vi "Profile Descriptor.vi"(10 "Profile":string[](array[string]), 11 "Descriptor":string) -> (3 "Flavoured Descriptor":string)   [LabVIEW 2015]
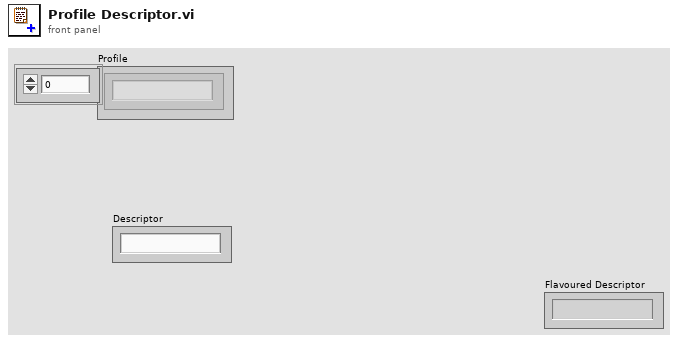
[diagram p1: front panel]
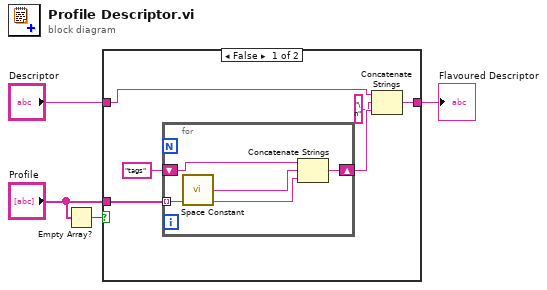
[diagram p0: block diagram]
diagram:
  n1 = Empty Array?(array="Profile") -> (empty?=w1:bool)
  n2 = case shown="False" w1 {
    tunnel: "Profile" -> [w10 _]
    tunnel: "Descriptor" -> [w9 w15]
    tunnel: [w8 w15] -> w3
    frame False {
      n3 = for {
        tunnel: w10 -> [w11] mode=indexing
        shift-right: [w14] -> w7
        shift-left: "tags" -> [w13]
        n4 = call <vilib>:"Space Constant.vi"() -> ("String"=w12:string)
        n5 = Concatenate Strings(w13, w12, w11) -> (w14:string)
      }
      n6 = Concatenate Strings(w9, "\n" ("string"), w7) -> (w8:string)
    }
    frame True {
    }
  }
  "Flavoured Descriptor" <- w3
